vi "thermo_build_tag.vi"(2 "capital":bool, 3 "index":u8, 4 "tag in":string, 5 "tag prefix":string) -> (0 "tag out":string, 1 "merged tag out":string)   [LabVIEW 2020]
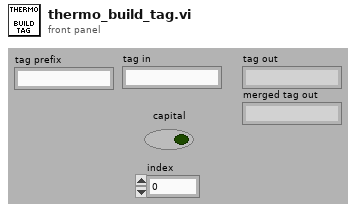
[diagram p1: front panel]
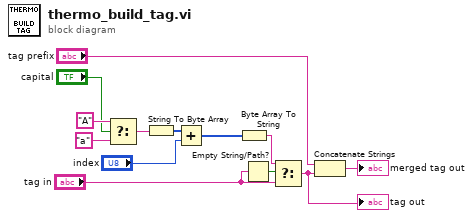
[diagram p0: block diagram]
diagram:
  n1 = Select(t="A" ("string"), s="capital", f="a") -> (s? t:f=w10:string)
  n2 = String To Byte Array(string=w10) -> (unsigned byte array=w9:u8[])
  n3 = Add(x=w9, y="index") -> (x+y=w8:u8[])
  n4 = Byte Array To String(unsigned byte array=w8) -> (string=w12:string)
  n5 = Empty String/Path?(string/path="tag in") -> (empty?=w13:bool)
  n6 = Select(t=w12, s=w13, f="tag in") -> (s? t:f=w11:string)
  "tag out" <- w11
  n7 = Concatenate Strings("tag prefix", w11) -> (→"merged tag out":string)
